vi "Initialization_HH.vi"(0 "Mode":i32=2 min=0 max=3 step=1) -> (1 "Initialisation Error":bool, 2 "Deviceindex":i32, 3 "DLL Version":string, 4 "Initialization Status":string, 5 "Serial[8]":string="**********")   [LabVIEW 2009]
uses:
  hhlib.dll
panel:
  out "Returncode HH_GetHardwareVersion":i32
  in  "String3[16]":string="*****************"
  in  "String4[8]":string="**********"
  out "Returncode HH_Initialize":i32
  in  "String2[8]":string="**********"
  in  "String1[8]":string="**********"
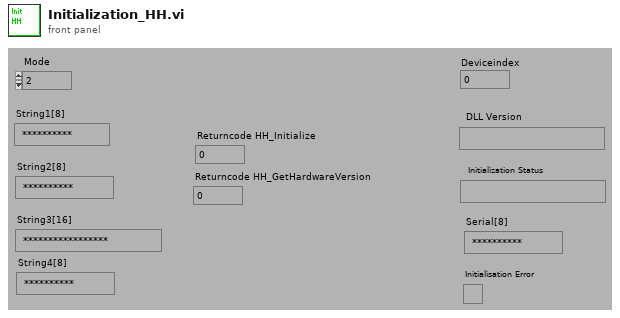
[diagram p1: front panel]
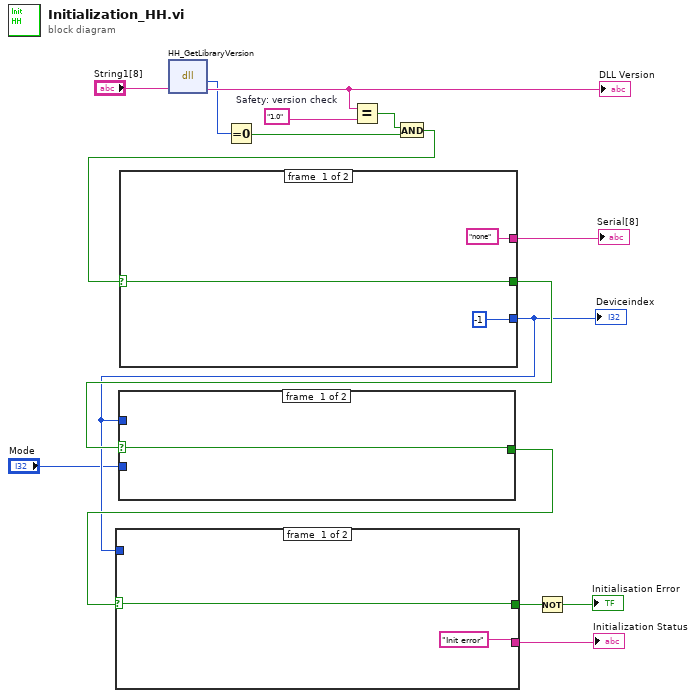
[diagram p0: block diagram]
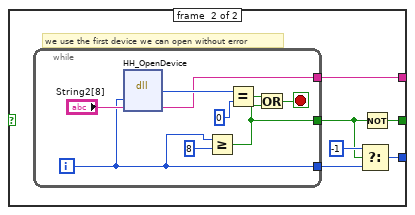
[diagram p2: hidden frame]
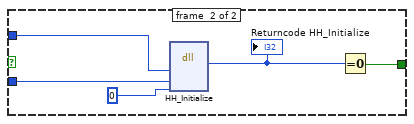
[diagram p3: hidden frame]
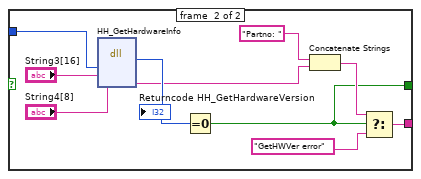
[diagram p4: hidden frame]
diagram:
  w13 = "1.0"  # Safety: version check
  n1 = dll-call lib="C:/Programme/Anwendungen/DAQLinescan_HH/hhlib.dll" fn="HH_GetLibraryVersion"("Version"="String1[8]") -> (w10:i32, "Version"=w14:string)  [unwired: 3 in, 2 out]
  "DLL Version" <- w14
  n2 = Equal To 0?(x=w10) -> (x = 0?=w11:bool)
  n3 = Equal?(x=w14, y=w13) -> (x = y?=w12:bool)
  n4 = And(x=w12, y=w11) -> (x .and. y?=w6:bool)
  n5 = case shown="True" w6 {
    selector: w6 -> [w18 _]
    tunnel: [w18 w20] -> w7
    tunnel: [-1 w23] -> w2
    tunnel: ["none" w19] -> w3
    frame #0 {
    }
    frame #1 {
      # "we use the first device we can open without error"
      n6 = while {
        tunnel: [w25] -> w19
        tunnel: [w29] -> w24
        tunnel: [w27] -> w21
        i -> [w29]
        stop <- w26 stop-if-true
        n7 = dll-call lib="C:/Programme/Anwendungen/DAQLinescan_HH/hhlib.dll" fn="HH_OpenDevice"("devidx"=w29, "serial"="String2[8]") -> (w31:i32, "serial"=w25:string)  [unwired: 4 in, 2 out]
        n8 = Greater Or Equal?(x=w29, y=8) -> (x >= y?=w27:bool)
        n9 = Equal?(x=w31, y=0) -> (x = y?=w28:bool)
        n10 = Or(x=w28, y=w27) -> (x .or. y?=w26:bool)
      }
      n11 = Select(t=-1, s=w21, f=w24) -> (s? t:f=w23:i32)
      n12 = Not(x=w21) -> (.not. x?=w20:bool)
    }
  }
  "Deviceindex" <- w2
  "Serial[8]" <- w3
  n13 = case shown="True" w7 {
    selector: w7 -> [w34 _]
    tunnel: [w34 w38] -> w8
    tunnel: w2 -> [_ w37]
    tunnel: "Mode" -> [_ w36]
    frame #0 {
    }
    frame #1 {
      n14 = dll-call lib="C:/Programme/Anwendungen/DAQLinescan_HH/hhlib.dll" fn="HH_Initialize"("devidx"=w37, "mode"=w36, "refsrc"=0) -> (w39:i32)  [unwired: 6 in, 2 out]
      "Returncode HH_Initialize" <- w39
      n15 = Equal To 0?(x=w39) -> (x = 0?=w38:bool)
    }
  }
  n16 = case shown="True" w8 {
    selector: w8 -> [w40 _]
    tunnel: ["Init error" w47] -> w4
    tunnel: [w40 w46] -> w9
    tunnel: w2 -> [_ w45]
    frame #0 {
    }
    frame #1 {
      n17 = dll-call lib="C:/Programme/Anwendungen/DAQLinescan_HH/hhlib.dll" fn="HH_GetHardwareInfo" label="HH_GetHardwareVersion"("devidx"=w45, "Model"="String3[16]", "Partno"="String4[8]") -> (w49:i32, "Partno"=w42:string)  [unwired: 5 in, 2 out]
      "Returncode HH_GetHardwareVersion" <- w49
      n18 = Equal To 0?(x=w49) -> (x = 0?=w46:bool)
      n19 = Concatenate Strings("Partno: ", w42) -> (w51:string)
      n20 = Select(t=w51, s=w46, f="GetHWVer error") -> (s? t:f=w47:string)
    }
  }
  "Initialization Status" <- w4
  n21 = Not(x=w9) -> (.not. x?=→"Initialisation Error":bool)
